vi "subSearchForAddons.vi"() -> (3 "Addons":path[](array[path]))   [LabVIEW 2020, in "UserInterface.lvlib" / "UIManager.lvclass"]
uses:
  UIManager.lvclass
  <vilib>/Utility/LVLibp/NI_PackedLibraryUtility.lvlib
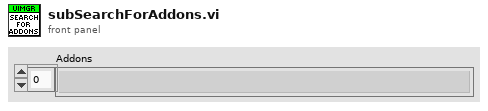
[diagram p1: front panel]
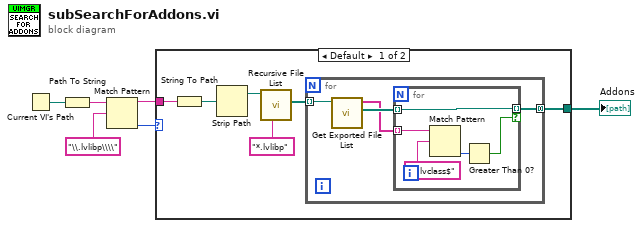
[diagram p0: block diagram]
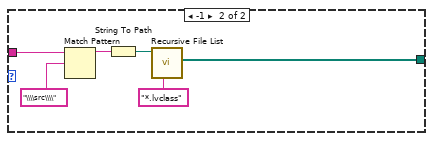
[diagram p2: hidden frame]
diagram:
  n1 = Current VI's Path() -> (path=w4:path)
  n2 = Path To String(path=w4) -> (string=w5:string)
  n3 = Match Pattern(string=w5, regular expression="\\.lvlibp\\\\") -> (before substring=w2:string, offset past match=w3:i32)  [unwired: 1 in, 2 out]
  n4 = case shown="Default" w3 {
    tunnel: w2 -> [w12 w25]
    tunnel: [w7 w22] -> w1
    frame Default {
      n5 = String To Path(string=w12) -> (path=w11:path)
      n6 = Strip Path(path=w11) -> (stripped path=w9:path)  [unwired: 1 out]
      n7 = call <vilib>:"Recursive File List.vi"("pattern"="*.lvlibp", "Folder Path"=w9) -> ("All Files in Dir"=w8:path[])  [unwired: 5 in, 4 out]
      n8 = for {
        tunnel: w8 -> [w16] mode=indexing
        tunnel: [w13] -> w7 mode=concatenating
        n9 = call <vilib>:"Get Exported File List.vi"("packed library path"=w16) -> ("paths"=w15:path[], "qualified names"=w14:string[])  [unwired: 8 in, 1 out]
        n10 = for {
          tunnel: w14 -> [w21] mode=indexing
          tunnel: w15 -> [w18] mode=indexing
          tunnel: [w18] -> w13 mode=indexing if=w17
          n11 = Match Pattern(string=w21, regular expression="\\.lvclass$") -> (offset past match=w19:i32)  [unwired: 1 in, 3 out]
          n12 = Greater Than 0?(x=w19) -> (x > 0?=w17:bool)
        }
      }
    }
    frame -1 {
      n13 = Match Pattern(string=w25, regular expression="\\\\src\\\\") -> (before substring=w24:string)  [unwired: 1 in, 3 out]
      n14 = String To Path(string=w24) -> (path=w23:path)
      n15 = call <vilib>:"Recursive File List.vi"("pattern"="*.lvclass", "Folder Path"=w23) -> ("All Files in Dir"=w22:path[])  [unwired: 5 in, 4 out]
    }
  }
  "Addons" <- w1
